vi "Untitled 6.vi"() -> ()   [LabVIEW 2009]
uses:
  <vilib>/sound/lvsound.llb/Sound Format.ctl
  <vilib>/Analysis/baseanly.llb/Scale 1D.vi
  <vilib>/measure/matone.llb/SINAD Analyzer 1 Chan.vi
  <vilib>/measure/NI_MAPro.lvlib
  <vilib>/Analysis/NI_AALBase.lvlib
panel:
  in  "volume":u16=65535
  out "SINAD (dB)":dbl(slide) scale=0.01..50.0
  out "detected fundamental\nfrequency":dbl format="%.6f"
  out "stereo 16-bit":waveform(dbl)[](graph)
  in  "STOP":bool
  out "error out":errorcluster
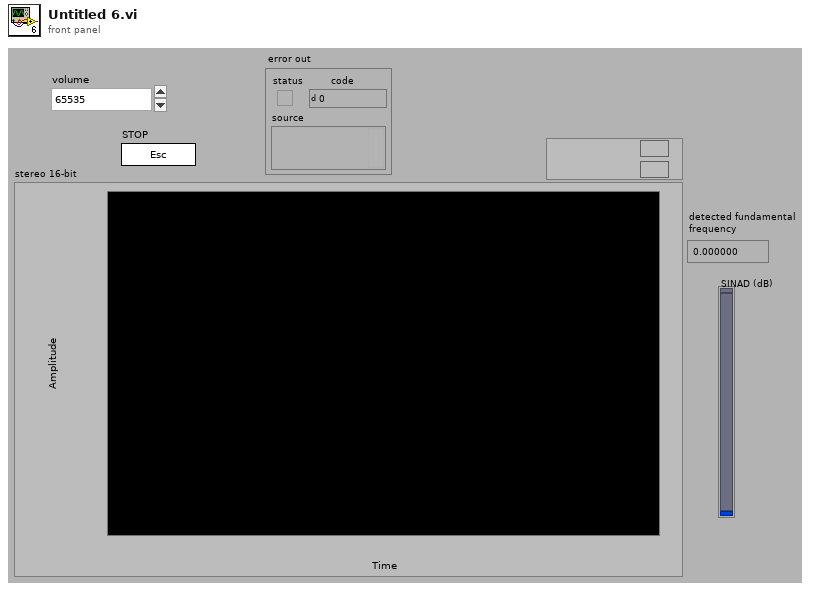
[diagram p1: front panel]
types:
  T1 = typedef "Sound Format.ctl" = cluster{"sound quality":enum16{"mono", "stereo"}, "rate":enum16{"11025", "22050", "44100", "8000"}, "bits per sample":enum16{"8 bit", "16 bit"}}
  T2 = enum16{"none", "input signal", "fundamental signal", "residual signal"}
  T3 = cluster{"exported time signal":waveform(dbl), "exported spectrum (dB)":cluster{"f0":dbl, "df":dbl, "dB Spectrum (Hann)":dbl[]}}
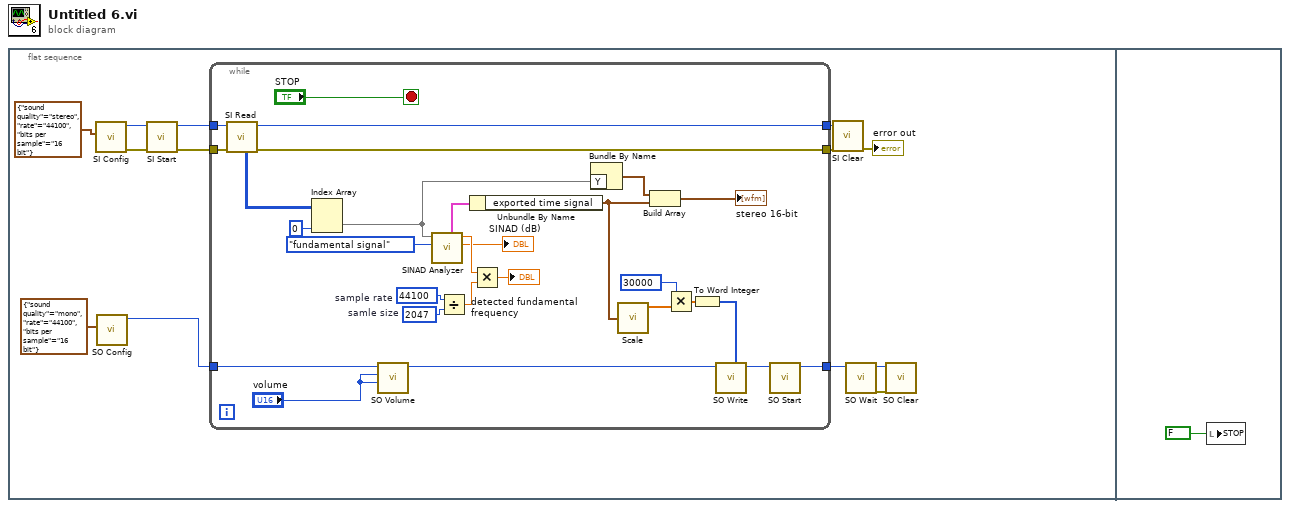
[diagram p0: block diagram]
diagram:
  n1 = flat-sequence {
    frame #0 {
      n2 = call <vilib>:"SI Config.vi"("sound format"=T1 {"sound quality"=enum."stereo", "rate"=enum."44100", "bits per sample"=enum."16 bit"}) -> ("error out"=w12:errorcluster, "task ID out"=w13:u32)  [unwired: 9 in]
      n3 = call <vilib>:"SO Config.vi"("sound format"=T1 {"sound quality"=enum."mono", "rate"=enum."44100", "bits per sample"=enum."16 bit"}) -> ("task ID out"=w1:u32)  [unwired: 9 in, 1 out]
      n4 = call <vilib>:"SI Start.vi"("error in (no error)"=w12, "task ID in"=w13) -> ("error out"=w7:errorcluster, "task ID out"=w8:u32)  [unwired: 8 in]
      n5 = while {
        tunnel: [w41] -> w11
        tunnel: [w40] -> w10
        tunnel: w8 -> [w39]
        tunnel: w7 -> [w38]
        tunnel: w1 -> [w22]
        tunnel: [w14] -> w5
        stop <- "STOP" stop-if-true
        w31 = 44100  # sample rate
        w32 = 2047  # samle size
        n6 = call <vilib>:"SI Read.vi"("error in (no error)"=w38, "task ID in"=w39) -> ("error out"=w41:errorcluster, "task ID out"=w40:u32, "stereo 16-bit"=w35:i16[][])  [unwired: 4 in, 3 out]
        n7 = Index Array(array=w35, index (col)=0 ("disabled index (col)")) -> (element=w26:i16[])  [unwired: 1 in]
        n8 = call <vilib>:"SO Volume.vi"("right channel"="volume", "left channel"="volume", "task ID in"=w22) -> ("task ID out"=w16:u32)  [unwired: 7 in, 1 out]
        n9 = call-poly <vilib>:"SINAD Analyzer.vi"("export signals"=T2."fundamental signal", "signal in"=w26) -> ("SINAD (dB)"=→"SINAD (dB)":dbl, "detected fundamental\nfrequency"=w33:dbl, "exported signals"=w27:T3)  [unwired: 4 in, 3 out]
        n10 = Divide(x=w31, y=w32) -> (x/y=w34:dbl)
        n11 = Unbundle By Name(w27) -> ("exported time signal"=w21:waveform(dbl))
        n12 = Multiply(x=w33, y=w34) -> (x*y=→"detected fundamental\nfrequency":dbl)
        n13 = Bundle By Name("Y"=w26) -> (w30:waveform(i16))  [unwired: 1 in]
        n14 = call-poly <vilib>:"Scale.vi"("X"=w21) -> ("Y=(X-offset)/scale"=w20:dbl[])  [unwired: 3 out]
        n15 = Build Array(w30, w21) -> (→"stereo 16-bit":waveform(dbl)[])
        n16 = Multiply(x=i16 30000, y=w20) -> (x*y=w18:dbl[])
        n17 = To Word Integer(number=w18) -> (16bit integer=w17:i16[])
        n18 = call <vilib>:"SO Write.vi"("mono 16-bit"=w17, "task ID in"=w16) -> ("task ID out"=w15:u32)  [unwired: 8 in, 1 out]
        n19 = call <vilib>:"SO Start.vi"("task ID in"=w15) -> ("task ID out"=w14:u32)  [unwired: 9 in, 1 out]
      }
      n20 = call <vilib>:"SI Clear.vi"("error in (no error)"=w11, "task ID in"=w10) -> ("error out"=→"error out":errorcluster)  [unwired: 9 in]
      n21 = call <vilib>:"SO Wait.vi"("task ID in"=w5) -> ("error out"=w4:errorcluster, "task ID out"=w3:u32)  [unwired: 9 in]
      n22 = call <vilib>:"SO Clear.vi"("error in (no error)"=w4, "task ID in"=w3) -> ()  [unwired: 9 in, 1 out]
    }
    frame #1 {
      n23 = local write "STOP"(FALSE ("Boolean")) -> ()
    }
  }
